vi "Handle Data.vi"(8 "error in (no error)":errorcluster, 10 "Data":T1, 11 "SubscribedDataHandler in":refnum<class "SubscribedDataHandler.lvclass">) -> (0 "error out":errorcluster)   [LabVIEW 2020, in "Vecto.lvlib" / "SubscribedDataHandler.lvclass"]
uses:
  SubscribedDataHandler.lvclass
  Subscribed Data.ctl
  Vecto.lvlib
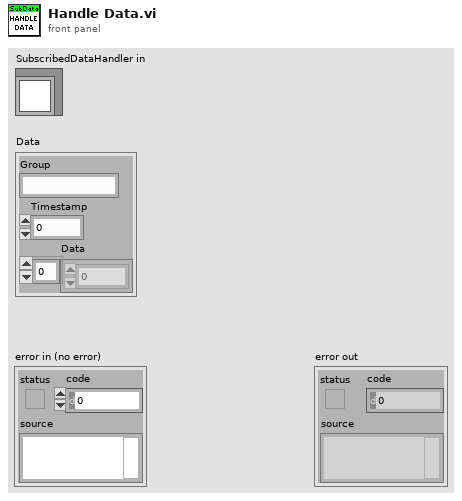
[diagram p1: front panel]
types:
  T1 = typedef "Vecto.lvlib/Subscribed Data.ctl" = cluster{"Group":string, "Timestamp":dbl, "Data":dbl[]}
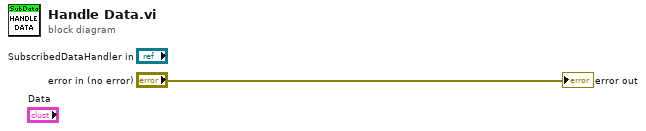
[diagram p0: block diagram]
diagram:
  "error out" <- "error in (no error)"
